vi "禹山浊度校准.vi"() -> ()   [LabVIEW 2016, in "斯坦道多参数.lvlib"]
uses:
  <vilib>/Utility/miscctls.llb/LVPointTypeDef.ctl
  <vilib>/Analysis/NI_AALBase.lvlib
  <vilib>/Analysis/NI_AALPro.lvlib
  <vilib>/Utility/config.llb/NI_LVConfig.lvlib
panel:
  out "第二点校准值":dbl
  out "第一点校准值":dbl
  out "最小值":sgl format="%.2g"
  out "最大值":sgl format="%.2g"
  in  "校准停止":bool
  in  "校准模式":enum16{"两点校准", "单点校准"}(ring)
  in  "标液2":dbl
  in  "标液1":dbl
  out "波形图表":sgl(graph) caption="历史曲线"
  out "温度测量值":dbl caption="温度"
  out "变异系数":dbl format="%.6g"
  out "standard deviation":dbl caption="标准差" format="%0.2f"
  out "mean":dbl caption="均值" format="%0.2f"
  out "提示":string
  in  "校准启动":bool
  out "测试值":dbl
  out "电极斜率":dbl
  out "电极零点":dbl
  # "浊度电极设定"
  # "℃"
  # "NTU"
  # "请选择校准模式:"
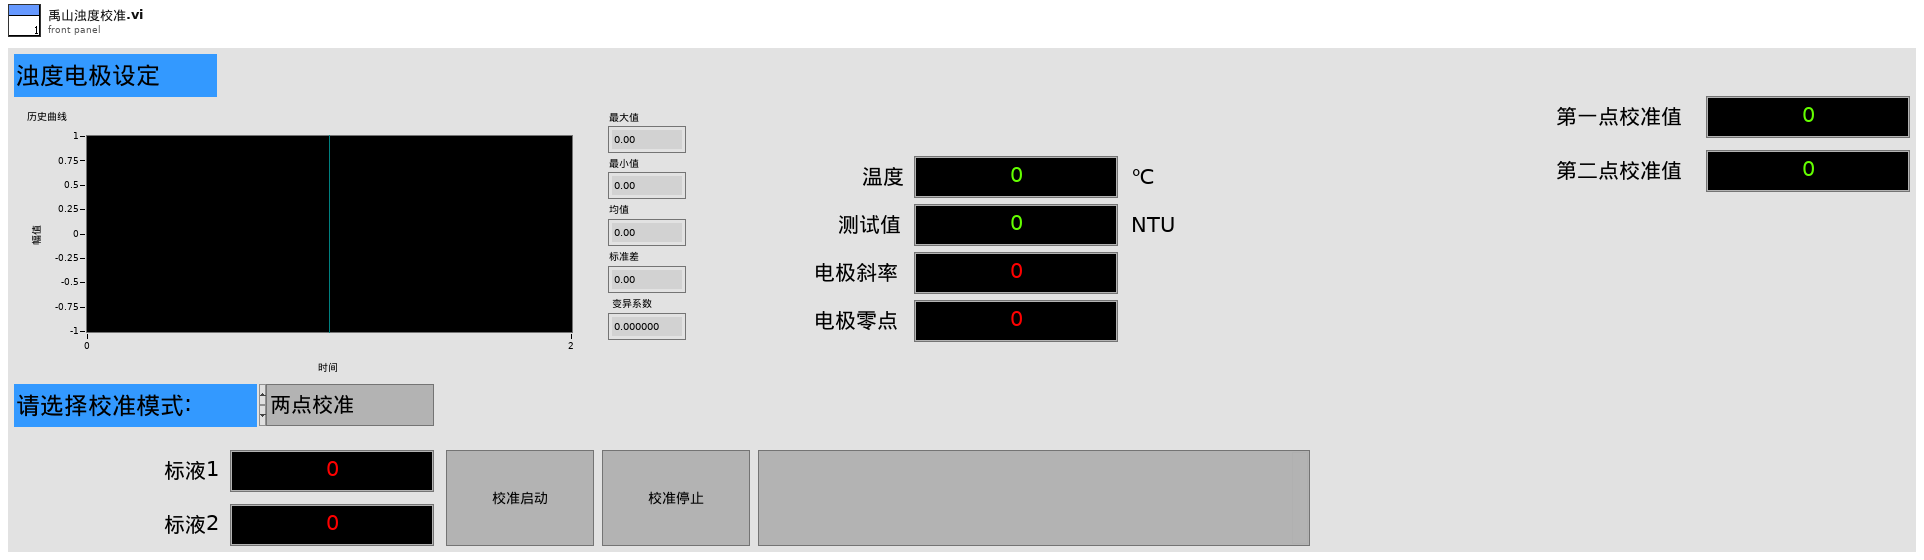
[diagram p1: front panel]
types:
  T1 = typedef "斯坦道多参数.lvlib/校准步骤.ctl" = enum16{"待机", "放置第一点标液", "第一点校准启动", "第一点校准写入", "第一点校准失败", "放置第二点标液", "第二点校准启动", "第二点校准写入", "第二点校准失败", "校准结果写入", "校准结束"}
  T2 = typedef "LVPointTypeDef.ctl" = cluster{"Horizontal":i16, "Vertical":i16}
  T3 = typedef "NI_LVConfig.lvlib/Config Data RefNum.ctl" = refnum<k1>
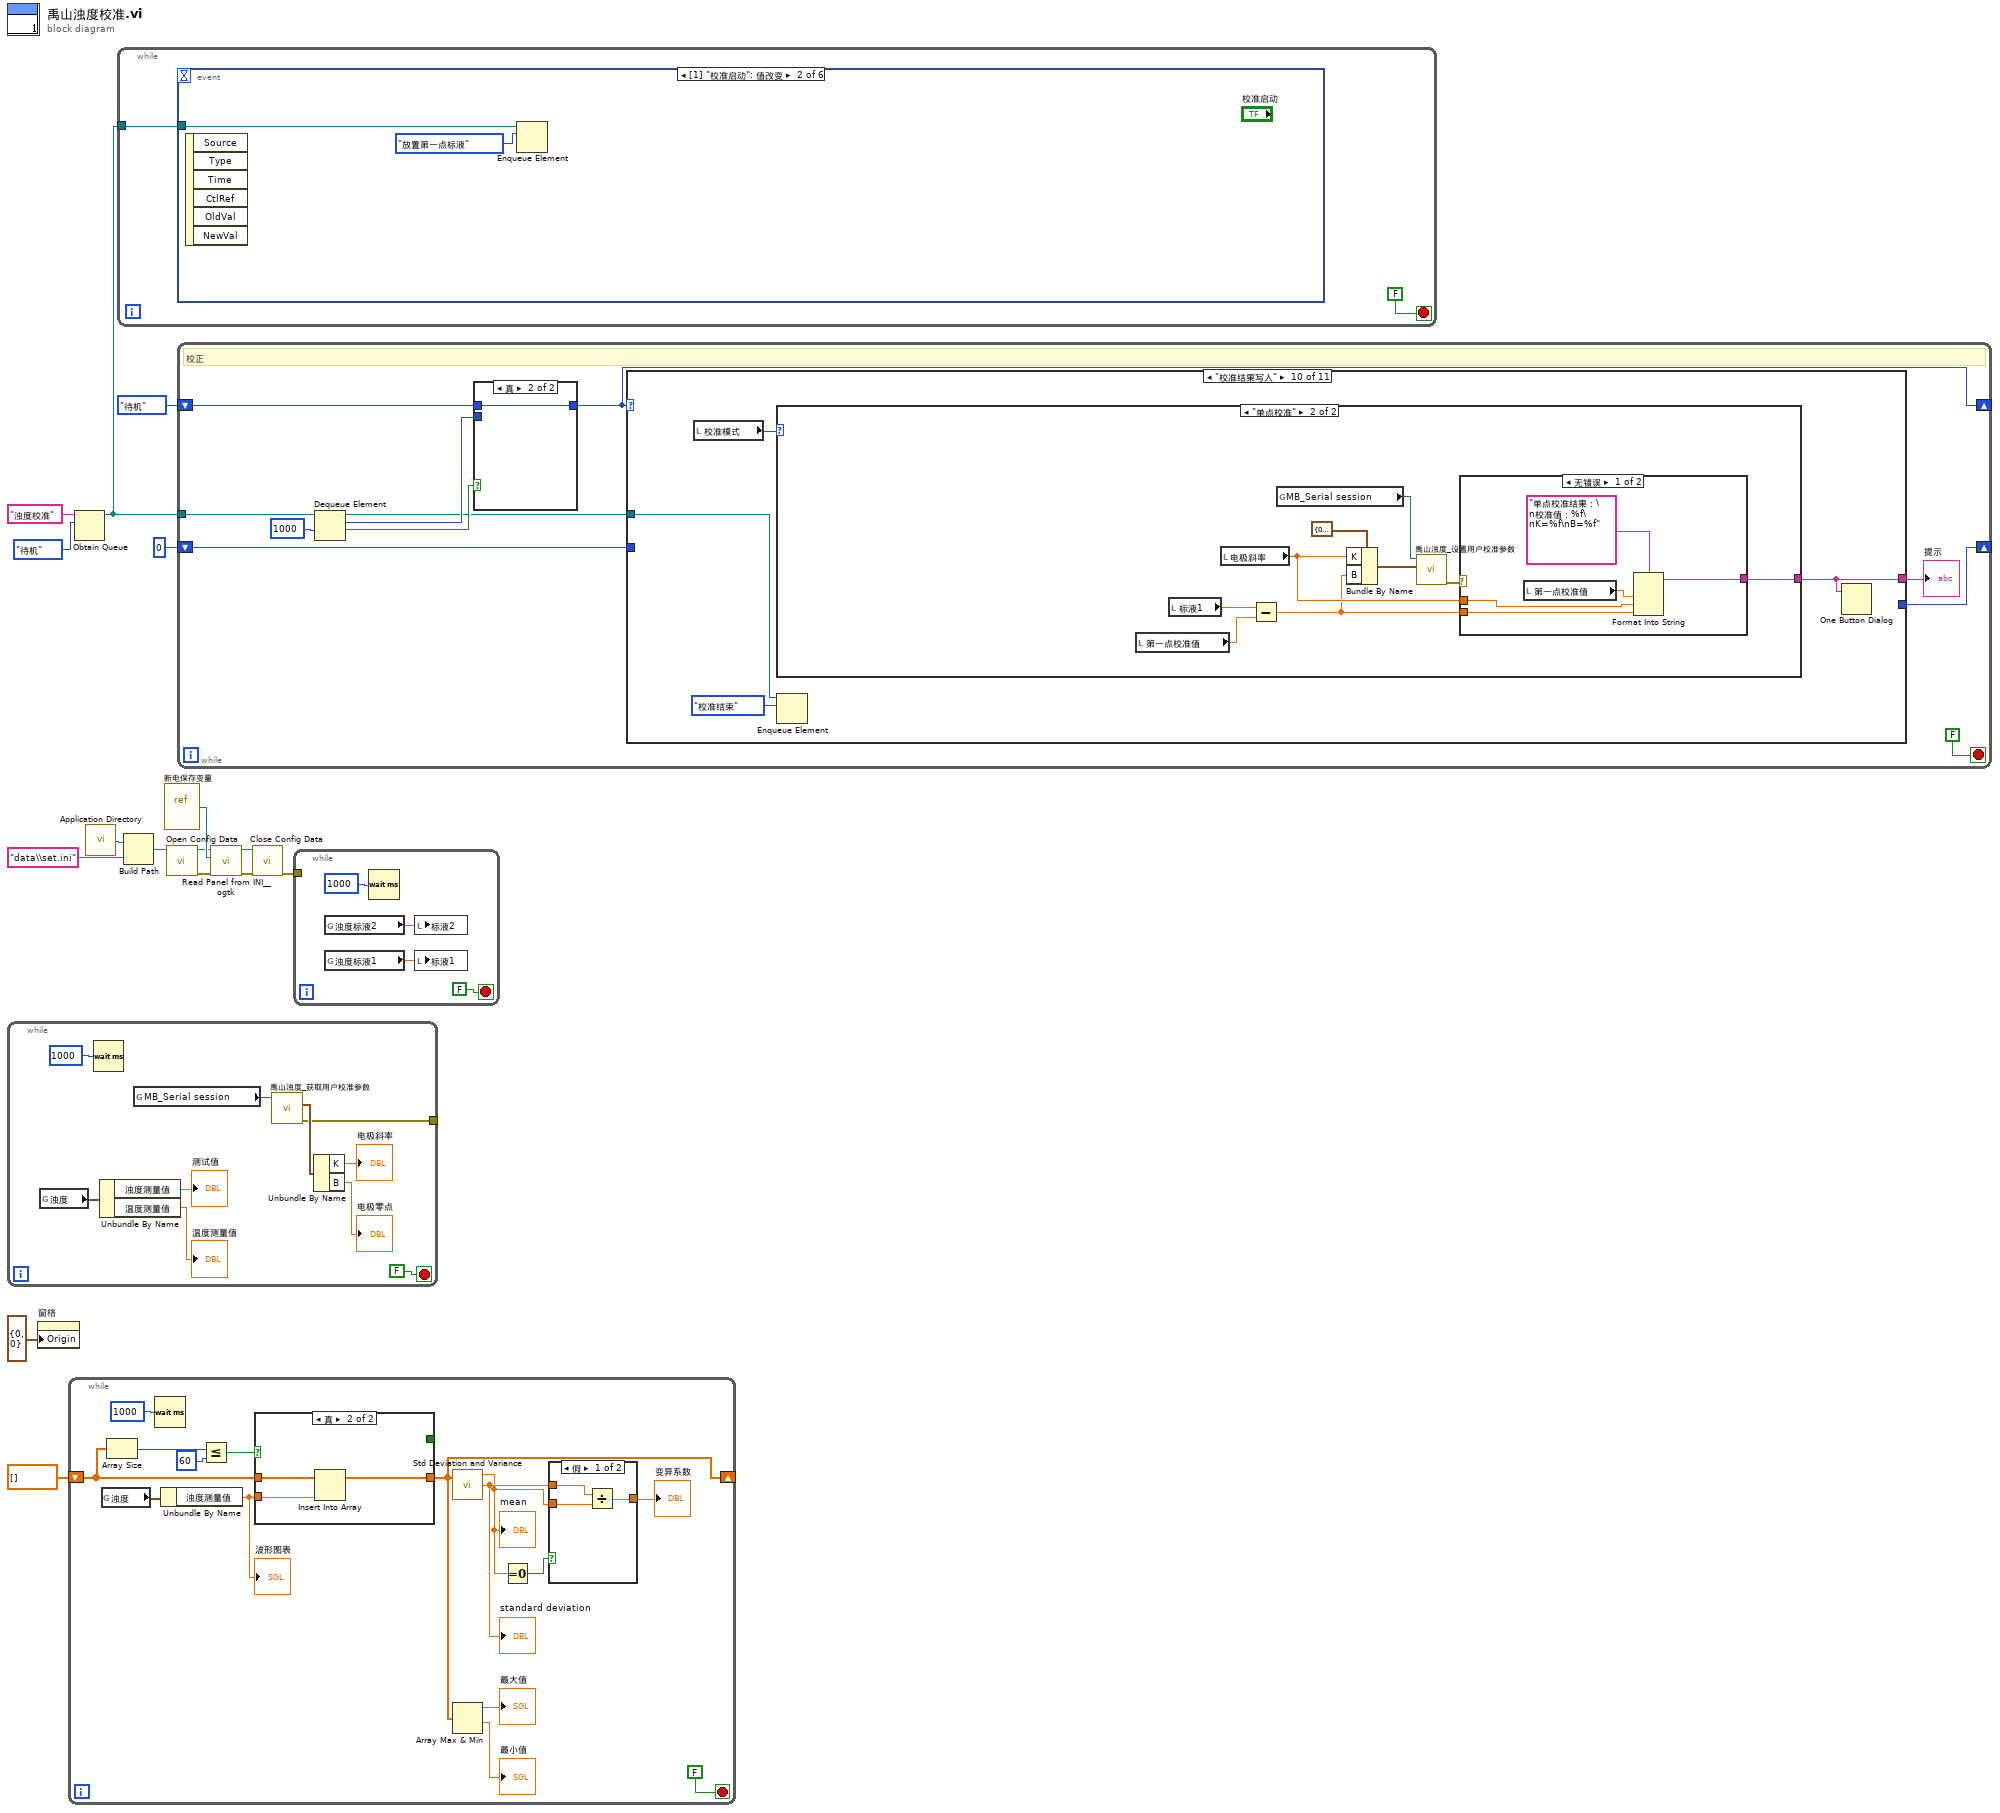
[diagram p0: block diagram]
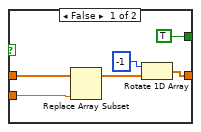
[diagram p3: hidden frame]
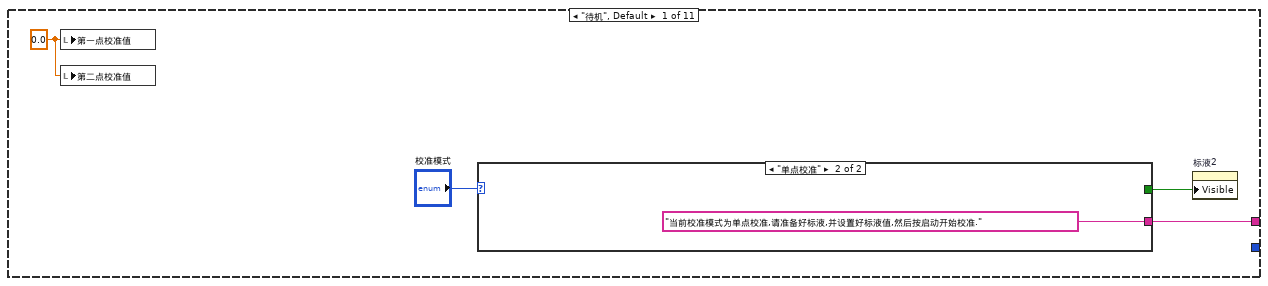
[diagram p5: hidden frame]
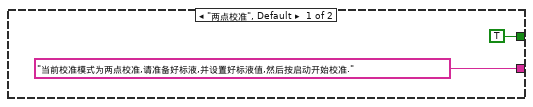
[diagram p6: hidden frame]
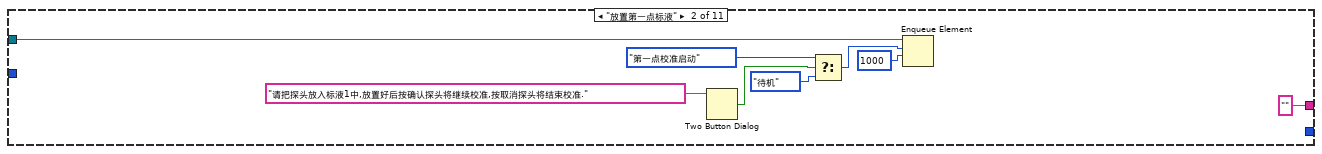
[diagram p7: hidden frame]
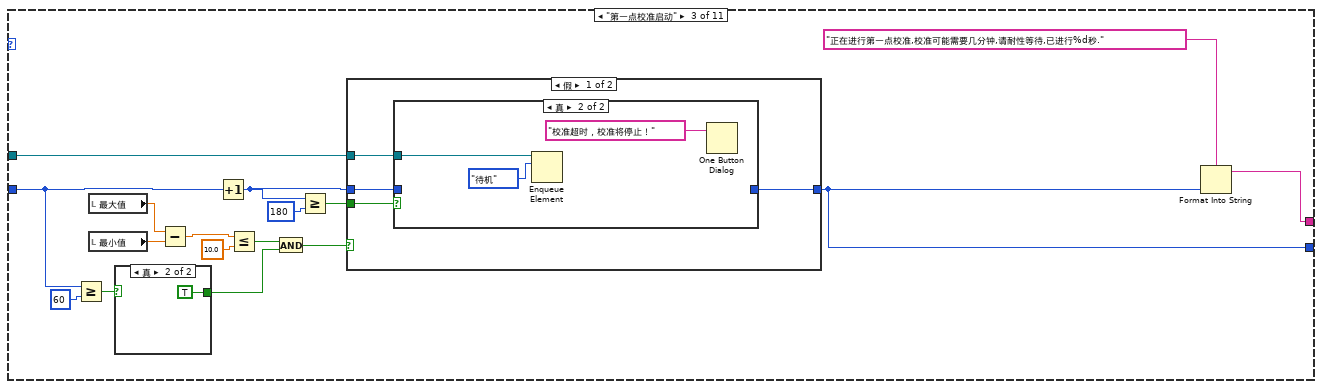
[diagram p8: hidden frame]
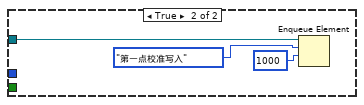
[diagram p10: hidden frame]
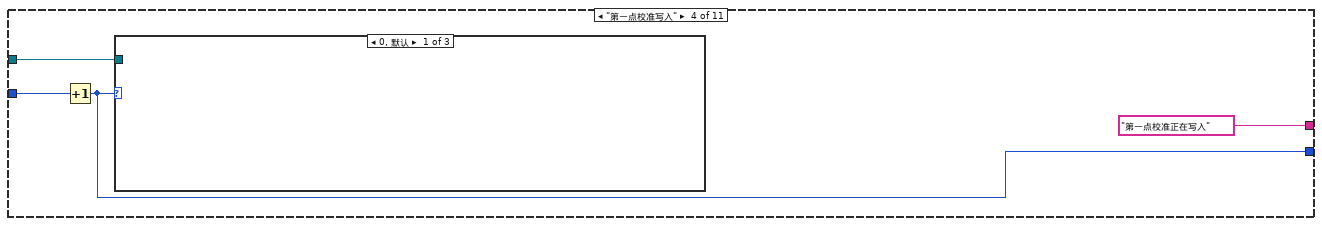
[diagram p12: hidden frame]
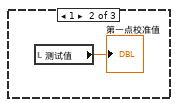
[diagram p13: hidden frame]
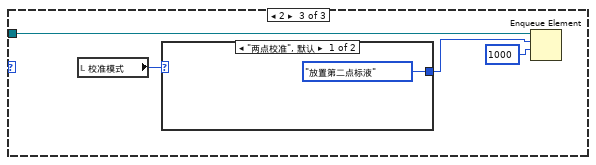
[diagram p14: hidden frame]
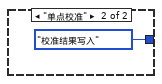
[diagram p15: hidden frame]
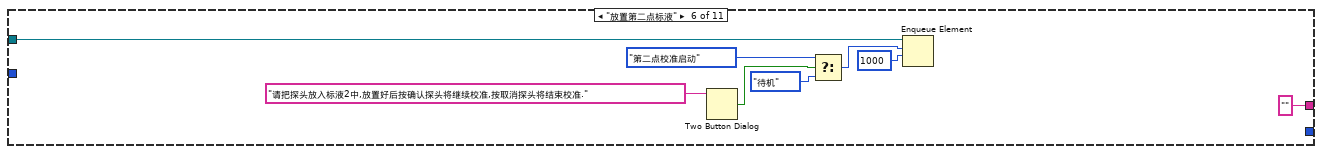
[diagram p17: hidden frame]
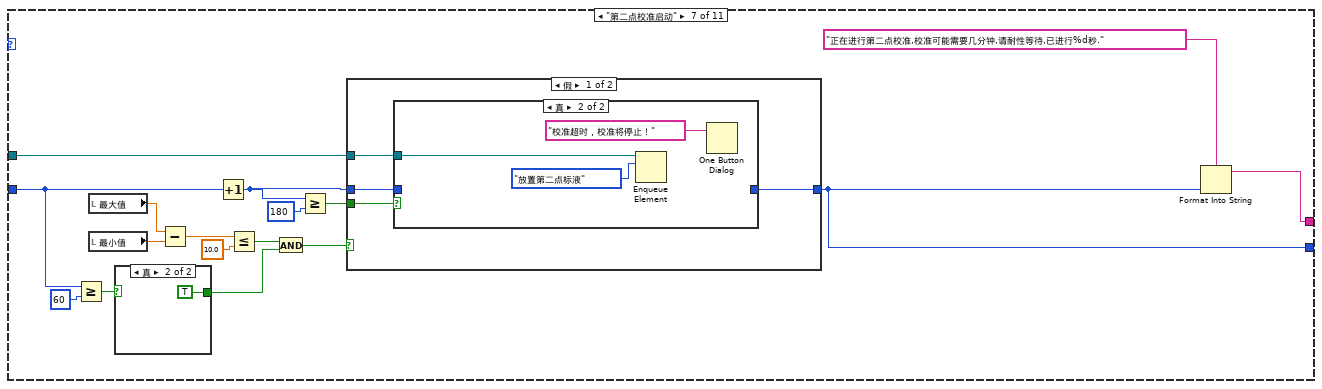
[diagram p18: hidden frame]
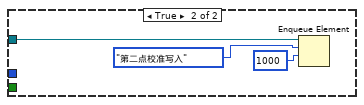
[diagram p20: hidden frame]
diagram:
  n1 = while {
    tunnel: [w21] -> _
    stop <- FALSE stop-if-true
    n2 = global read "禹山过程全局变量.vi" "浊度"() -> (w18:cluster{"温度测量值":sgl, "浊度测量值":sgl})
    n3 = Wait (ms)(milliseconds to wait=u32 1000 ("等待时间（毫秒）")) -> ()  [unwired: 1 out]
    n4 = Unbundle By Name(w18) -> ("浊度测量值"=→"测试值":sgl, "温度测量值"=→"温度测量值":sgl)
    n5 = global read "多参数全局变量.vi" "MB_Serial session"() -> (w17:refnum<class "MB_Master_Serial.lvclass">)
    n6 = call "禹山浊度_获取用户校准参数.vi"("MB_Serial session in"=w17) -> ("error out"=w21:errorcluster, "输出值"=w24:cluster{"K":sgl, "B":sgl})  [unwired: 8 in, 1 out]
    n7 = Unbundle By Name(w24) -> ("K"=→"电极斜率":sgl, "B"=→"电极零点":sgl)
  }
  n8 = property on="窗格" class="Pane"("Origin"=T2 {"Horizontal"=0, "Vertical"=0} ("原点")) -> ()  [unwired: 2 in, 2 out]
  n9 = while {
    shift-right: [w29] -> _
    shift-left: sgl[] [] -> [w37]
    stop <- FALSE stop-if-true
    n10 = global read "禹山过程全局变量.vi" "浊度"() -> (w31:cluster{"温度测量值":sgl, "浊度测量值":sgl})
    n11 = Array Size(array=w37) -> (size(s)=w39:i32)
    n12 = Wait (ms)(milliseconds to wait=u32 1000 ("等待时间（毫秒）")) -> ()  [unwired: 1 out]
    n13 = Unbundle By Name(w31) -> ("浊度测量值"=w30:sgl)
    "波形图表" <- w30
    n14 = Less Or Equal?(x=w39, y=60) -> (x <= y?=w38:bool)
    n15 = case shown="真" w38 {
      tunnel: w37 -> [w50 w53]
      tunnel: w30 -> [w48 w52]
      tunnel: [w46 w51] -> w29
      tunnel: [TRUE _] -> _
      frame False {
        n16 = Replace Array Subset(array=w50, new element=w48) -> (w49:sgl[])  [unwired: 1 in]
        n17 = Rotate 1D Array(1:w49, 2:-1 ("n")) -> (0:w46:sgl[])
      }
      frame True {
        n18 = Insert Into Array(array=w53, new element=w52) -> (w51:sgl[])  [unwired: 1 in]
      }
    }
    n19 = call <vilib>:"Std Deviation and Variance.vi"("X"=w29) -> ("mean"=w32:dbl, "standard deviation"=w33:dbl)  [unwired: 1 in, 1 out]
    "standard deviation" <- w33
    "mean" <- w32
    n20 = Array Max & Min(array=w29) -> (max value=→"最大值":sgl, min value=→"最小值":sgl)  [unwired: 2 out]
    n21 = Equal To 0?(x=w32) -> (x = 0?=w36:bool)
    n22 = case shown="假" w36 {
      tunnel: w33 -> [w44 _]
      tunnel: [w43 _] -> w35
      tunnel: w32 -> [w42 _]
      frame False {
        n23 = Divide(x=w44, y=w42) -> (x/y=w43:dbl)
      }
      frame True {
      }
    }
    "变异系数" <- w35
  }
  n24 = Obtain Queue(name (unnamed)="浊度校准" ("名称（未命名）"), element data type=校准步骤."待机" ("枚举")) -> (queue out=w10:refnum<queue>)  [unwired: 3 in, 2 out]
  n25 = call <vilib>:"Application Directory.vi"() -> ("Application Directory"=w6:path)
  n26 = while {
    tunnel: w10 -> [w54]
    stop <- FALSE stop-if-true
    n27 = event shown="[1] \"校准启动\": 值改变" {
      selector: _ -> [_ _ _ _ _ _]
      dyn-events: _ -> [_ _ _ _ _ _]
      timeout: _ -> [_ _ _ _ _ _]
      tunnel: w54 -> [_ w57 w61 _ _ _]
      event Timeout {
        n28 = event-data() -> ()  [unwired: 1 in, 3 out]
      }
      event "校准启动": Value Change {
        n29 = event-data() -> ()  [unwired: 1 in, 6 out]
        n30 = Enqueue Element(queue=w57, element=校准步骤."放置第一点标液" ("元素")) -> ()  [unwired: 2 in, 3 out]
      }
      event "校准停止": Value Change {
        n31 = event-data() -> ()  [unwired: 1 in, 6 out]
        n32 = Flush Queue(queue=w61) -> (queue out=w58:refnum<queue>)  [unwired: 1 in, 2 out]
        n33 = Enqueue Element(queue=w58, element=校准步骤."待机" ("元素"), timeout in ms (-1)=1000 ("超时毫秒(-1)")) -> ()  [unwired: 1 in, 3 out]
      }
      event "电极零点", "电极斜率", "标液1", "标液2": Mouse Down {
        n34 = event-data() -> ("CtlRef"=w62:refnum<vi>)  [unwired: 1 in, 7 out]
        n35 = property class="DigNum (严格)"(reference=w62) -> (reference out=w63:refnum<vi>, "Value"=w64:dbl)  [unwired: 1 in, 1 out]
        n36 = call "数字键盘.vi"("OldNumber"=w64) -> ("NewNumber"=w65:sgl)
        n37 = property class="DigNum (严格)"(reference=w63, "Val(Sgnl)"=w65) -> ()  [unwired: 1 in, 2 out]
      }
      event "电极零点", "电极斜率": Value Change {
        n38 = event-data() -> ()  [unwired: 1 in, 6 out]
        n39 = local read "电极斜率"() -> (w68:dbl)
        n40 = local read "电极零点"() -> (w67:dbl)
        n41 = global read "多参数全局变量.vi" "MB_Serial session"() -> (w66:refnum<class "MB_Master_Serial.lvclass">)
        n42 = Bundle By Name(cluster=cluster{"K":sgl, "B":sgl} {"K"=0.0, "B"=0.0} ("用户校准参数"), "K"=w68, "B"=w67) -> (w69:cluster{"K":sgl, "B":sgl})
        n43 = call "禹山浊度_设置用户校准参数.vi"("用户校准参数"=w69, "MB_Serial session in"=w66) -> ()  [unwired: 8 in, 2 out]
      }
      event "标液1", "标液2": Value Change {
        n44 = event-data() -> ()  [unwired: 1 in, 6 out]
        n45 = flat-sequence {
          frame #0 {
            n46 = global write "断电保存变量.vi" "浊度标液2"("标液2") -> ()
            n47 = global write "断电保存变量.vi" "浊度标液1"("标液1") -> ()
          }
          frame #1 {
            n48 = call <vilib>:"Application Directory.vi"() -> ("Application Directory"=w82:path)
            n49 = Build Path(base path=w82, name or relative path="data\\set.ini" ("名称或相对路径")) -> (appended path=w81:path)
            n50 = call <vilib>:"Open Config Data.vi"("configuration file path"=w81) -> ("error out"=w85:errorcluster, "refnum"=w86:T3)  [unwired: 8 in, 1 out]
            n51 = vi-ref "断电保存变量.vi"() -> (w79:refnum<vi>)
            n52 = call <userlib>:"Write Panel to INI__ogtk.vi"("error in (no error)"=w85, "VI ref"=w79, "refnum"=w86) -> ("error out"=w83:errorcluster, "refnum out"=w84:T3)  [unwired: 7 in]
            n53 = call <vilib>:"Close Config Data.vi"("error in (no error)"=w83, "refnum"=w84) -> ("error out"=w75:errorcluster, "file path"=w76:path)  [unwired: 8 in]
            n54 = Open/Create/Replace File(file path (use dialog)=w76, error in=w75) -> (refnum out=w77:refnum<file>, error out=w78:errorcluster)  [unwired: 4 in, 1 out]
            n55 = Flush File(refnum=w77, error in=w78) -> (refnum out=w73:refnum<file>, error out=w74:errorcluster)
            n56 = Close File(refnum=w73, error in=w74) -> ()  [unwired: 2 out]
          }
        }
      }
    }
  }
  n57 = Build Path(base path=w6, name or relative path="data\\set.ini" ("名称或相对路径")) -> (appended path=w7:path)
  n58 = vi-ref "断电保存变量.vi"() -> (w9:refnum<vi>)
  n59 = call <vilib>:"Open Config Data.vi"("configuration file path"=w7) -> ("error out"=w3:errorcluster, "refnum"=w2:T3)  [unwired: 8 in, 1 out]
  n60 = while "While循环" {
    shift-right: [w88] -> _
    shift-left: 校准步骤."待机" ("枚举") -> [w89]
    shift-right: [w95] -> _
    shift-left: 0 -> [w96]
    tunnel: w10 -> [w93]
    stop <- FALSE stop-if-true
    # "校正"
    n61 = Dequeue Element(queue=w93, timeout in ms (-1)=1000 ("超时毫秒(-1)")) -> (queue out=w87:refnum<queue>, element=w90:T1, timed out?=w91:bool)  [unwired: 1 in, 1 out]
    n62 = case shown="真" w91 {
      tunnel: w90 -> [w98 _]
      tunnel: [w98 w99] -> w88
      tunnel: w89 -> [_ w99]
      frame False {
      }
      frame True {
      }
    }
    n63 = case shown="\"校准结果写入\"" w88 {
      tunnel: [w103 "" ("提示") w130 "第一点校准正在写入" ("提示") _ "" ("提示") w178 "第二点校准正在写入" ("提示") _ w203 w246] -> w94
      tunnel: w96 -> [_ _ w124 w146 _ _ w172 w194 _ _ _]
      tunnel: [_ _ w115 w145 _ _ w163 w193 _ _ _] -> w95
      tunnel: w87 -> [_ w113 w118 w144 _ w161 w166 w192 _ w202 _]
      frame "待机", Default {
        w100 = 0.0 ("第一点校准值")
        n64 = local write "第一点校准值"(w100) -> ()
        n65 = local write "第二点校准值"(w100) -> ()
        n66 = case shown="\"单点校准\"" "校准模式" {
          tunnel: ["当前校准模式为两点校准,请准备好标液,并设置好标液值,然后按启动开始校准." ("提示") "当前校准模式为单点校准,请准备好标液,并设置好标液值,然后按启动开始校准." ("提示")] -> w103
          tunnel: [TRUE ("可见") _] -> w101
          frame "两点校准", Default {
          }
          frame "单点校准" {
          }
        }
        n67 = property on="标液2" class="DigNum (严格)"("Visible"=w101) -> ()  [unwired: 2 in, 2 out]
      }
      frame "放置第一点标液" {
        n68 = Two Button Dialog(message="请把探头放入标液1中,放置好后按确认探头将继续校准,按取消探头将结束校准." ("消息")) -> (T button?=w111:bool)  [unwired: 2 in]
        n69 = Select(t=校准步骤."第一点校准启动" ("元素"), s=w111, f=校准步骤."待机" ("元素")) -> (s? t:f=w108:T1)
        n70 = Enqueue Element(queue=w113, element=w108, timeout in ms (-1)=1000 ("超时毫秒(-1)")) -> ()  [unwired: 1 in, 3 out]
      }
      frame "第一点校准启动" {
        n71 = Greater Or Equal?(x=w124, y=60) -> (x >= y?=w125:bool)
        n72 = local read "最大值"() -> (w121:sgl)
        n73 = local read "最小值"() -> (w122:sgl)
        n74 = case shown="真" w125 {
          tunnel: [_ TRUE] -> w123
          frame False {
          }
          frame True {
          }
        }
        n75 = Subtract(x=w121, y=w122) -> (x-y=w120:sgl)
        n76 = Increment(x=w124) -> (x+1=w116:i32)
        n77 = Less Or Equal?(x=w120, y=10.0) -> (x <= y?=w128:bool)
        n78 = And(x=w128, y=w123) -> (x .and. y?=w119:bool)
        n79 = Greater Or Equal?(x=w116, y=180) -> (x >= y?=w117:bool)
        n80 = case shown="假" w119 {
          tunnel: w118 -> [w134 w142]
          tunnel: w117 -> [w135 _]
          tunnel: w116 -> [w133 _]
          tunnel: [w132 _] -> w115
          frame False {
            n81 = case shown="真" w135 {
              tunnel: w134 -> [_ w139]
              tunnel: w133 -> [w136 _]
              tunnel: [w136 _] -> w132
              frame False {
              }
              frame True {
                n82 = Enqueue Element(queue=w139, element=校准步骤."待机" ("元素")) -> ()  [unwired: 2 in, 3 out]
                n83 = One Button Dialog(message="校准超时，校准将停止！" ("消息")) -> ()  [unwired: 1 in, 1 out]
              }
            }
          }
          frame True {
            n84 = Enqueue Element(queue=w142, element=校准步骤."第一点校准写入" ("元素"), timeout in ms (-1)=1000 ("超时毫秒(-1)")) -> ()  [unwired: 1 in, 3 out]
          }
        }
        n85 = Format Into String(format string="正在进行第一点校准,校准可能需要几分钟,请耐性等待,已进行%d秒." ("格式字符串"), w115) -> (resulting string=w130:string)  [unwired: 2 in, 1 out]
      }
      frame "第一点校准写入" {
        n86 = Increment(x=w146) -> (x+1=w145:i32)
        n87 = case shown="0, 默认" w145 {
          tunnel: w144 -> [_ _ w152]
          frame 0, Default {
          }
          frame 1 {
            n88 = local read "测试值"() -> (→"第一点校准值":dbl)
          }
          frame 2 {
            n89 = local read "校准模式"() -> (w151:enum16{"两点校准", "单点校准"})
            n90 = case shown="\"两点校准\", 默认" w151 {
              tunnel: [校准步骤."放置第二点标液" ("元素") 校准步骤."校准结果写入" ("元素")] -> w150
              frame "两点校准", Default {
              }
              frame "单点校准" {
              }
            }
            n91 = Enqueue Element(queue=w152, element=w150, timeout in ms (-1)=1000 ("超时毫秒(-1)")) -> ()  [unwired: 1 in, 3 out]
          }
        }
      }
      frame "第一点校准失败" {
      }
      frame "放置第二点标液" {
        n92 = Two Button Dialog(message="请把探头放入标液2中,放置好后按确认探头将继续校准,按取消探头将结束校准." ("消息")) -> (T button?=w159:bool)  [unwired: 2 in]
        n93 = Select(t=校准步骤."第二点校准启动" ("元素"), s=w159, f=校准步骤."待机" ("元素")) -> (s? t:f=w156:T1)
        n94 = Enqueue Element(queue=w161, element=w156, timeout in ms (-1)=1000 ("超时毫秒(-1)")) -> ()  [unwired: 1 in, 3 out]
      }
      frame "第二点校准启动" {
        n95 = Greater Or Equal?(x=w172, y=60) -> (x >= y?=w173:bool)
        n96 = local read "最大值"() -> (w169:sgl)
        n97 = local read "最小值"() -> (w170:sgl)
        n98 = case shown="真" w173 {
          tunnel: [_ TRUE] -> w171
          frame False {
          }
          frame True {
          }
        }
        n99 = Subtract(x=w169, y=w170) -> (x-y=w168:sgl)
        n100 = Increment(x=w172) -> (x+1=w164:i32)
        n101 = Less Or Equal?(x=w168, y=10.0) -> (x <= y?=w176:bool)
        n102 = And(x=w176, y=w171) -> (x .and. y?=w167:bool)
        n103 = Greater Or Equal?(x=w164, y=180) -> (x >= y?=w165:bool)
        n104 = case shown="假" w167 {
          tunnel: w166 -> [w182 w190]
          tunnel: w165 -> [w183 _]
          tunnel: w164 -> [w181 _]
          tunnel: [w180 _] -> w163
          frame False {
            n105 = case shown="真" w183 {
              tunnel: w182 -> [_ w187]
              tunnel: w181 -> [w184 _]
              tunnel: [w184 _] -> w180
              frame False {
              }
              frame True {
                n106 = Enqueue Element(queue=w187, element=校准步骤."放置第二点标液" ("元素")) -> ()  [unwired: 2 in, 3 out]
                n107 = One Button Dialog(message="校准超时，校准将停止！" ("消息")) -> ()  [unwired: 1 in, 1 out]
              }
            }
          }
          frame True {
            n108 = Enqueue Element(queue=w190, element=校准步骤."第二点校准写入" ("元素"), timeout in ms (-1)=1000 ("超时毫秒(-1)")) -> ()  [unwired: 1 in, 3 out]
          }
        }
        n109 = Format Into String(format string="正在进行第二点校准,校准可能需要几分钟,请耐性等待,已进行%d秒." ("格式字符串"), w163) -> (resulting string=w178:string)  [unwired: 2 in, 1 out]
      }
      frame "第二点校准写入" {
        n110 = Increment(x=w194) -> (x+1=w193:i32)
        n111 = case shown="2" w193 {
          tunnel: w192 -> [_ _ w199]
          frame 0, Default {
          }
          frame 1 {
            n112 = local read "测试值"() -> (→"第二点校准值":dbl)
          }
          frame 2 {
            n113 = Enqueue Element(queue=w199, element=校准步骤."校准结果写入" ("元素"), timeout in ms (-1)=1000 ("超时毫秒(-1)")) -> ()  [unwired: 1 in, 3 out]
          }
        }
      }
      frame "第二点校准失败" {
      }
      frame "校准结果写入" {
        n114 = local read "校准模式"() -> (w200:enum16{"两点校准", "单点校准"})
        n115 = case shown="\"单点校准\"" w200 {
          tunnel: [w211 w235] -> w203
          frame "两点校准", Default {
            n116 = local read "第一点校准值"() -> (w222:dbl)
            n117 = local read "第二点校准值"() -> (w221:dbl)
            n118 = local read "标液1"() -> (w219:dbl)
            n119 = local read "标液2"() -> (w218:dbl)
            n120 = Insert Into Array(array=dbl[] [] ("Weight"), new element #1=w219, new element #2=w218) -> (w217:dbl[])  [unwired: 1 in]
            n121 = Insert Into Array(array=dbl[] [] ("Weight"), new element #1=w222, new element #2=w221) -> (w216:dbl[])  [unwired: 1 in]
            n122 = local read "电极零点"() -> (w207:dbl)
            n123 = call <vilib>:"Linear Fit.vi"("Y"=w217, "X"=w216) -> ("slope"=w208:dbl, "intercept"=w205:dbl)  [unwired: 9 in, 3 out]
            n124 = local read "电极斜率"() -> (w210:dbl)
            n125 = Multiply(x=w208, y=w207) -> (x*y=w206:dbl)
            n126 = Multiply(x=w210, y=w208) -> (x*y=w209:dbl)
            n127 = Add(x=w206, y=w205) -> (x+y=w204:dbl)
            n128 = global read "多参数全局变量.vi" "MB_Serial session"() -> (w215:refnum<class "MB_Master_Serial.lvclass">)
            n129 = Bundle By Name(cluster=cluster{"K":sgl, "B":sgl} {"K"=0.0, "B"=0.0} ("用户校准参数"), "K"=w209, "B"=w204) -> (w214:cluster{"K":sgl, "B":sgl})
            n130 = call "禹山浊度_设置用户校准参数.vi"("用户校准参数"=w214, "MB_Serial session in"=w215) -> ("error out"=w212:errorcluster)  [unwired: 8 in, 1 out]
            n131 = case shown="无错误" w212 {
              tunnel: w209 -> [w226 _]
              tunnel: w204 -> [w225 _]
              tunnel: [w224 "校准失败"] -> w211
              frame No Error {
                n132 = local read "第一点校准值"() -> (w228:dbl)
                n133 = local read "第二点校准值"() -> (w229:dbl)
                n134 = Format Into String(format string="两点校准结果：\n第一点校准值：%f\n第二点校准值：%f\nK=%f\nB=%f" ("提示"), w228, w229, w226, w225) -> (resulting string=w224:string)  [unwired: 2 in, 1 out]
              }
              frame Error {
              }
            }
          }
          frame "单点校准" {
            n135 = local read "第一点校准值"() -> (w233:dbl)
            n136 = local read "标液1"() -> (w232:dbl)
            n137 = local read "电极斜率"() -> (w234:dbl)
            n138 = Subtract(x=w232, y=w233) -> (x-y=w231:dbl)
            n139 = global read "多参数全局变量.vi" "MB_Serial session"() -> (w239:refnum<class "MB_Master_Serial.lvclass">)
            n140 = Bundle By Name(cluster=cluster{"K":sgl, "B":sgl} {"K"=0.0, "B"=0.0} ("用户校准参数"), "K"=w234, "B"=w231) -> (w238:cluster{"K":sgl, "B":sgl})
            n141 = call "禹山浊度_设置用户校准参数.vi"("用户校准参数"=w238, "MB_Serial session in"=w239) -> ("error out"=w236:errorcluster)  [unwired: 8 in, 1 out]
            n142 = case shown="无错误" w236 {
              tunnel: w234 -> [w242 _]
              tunnel: w231 -> [w241 _]
              tunnel: [w240 "校准失败"] -> w235
              frame No Error {
                n143 = local read "第一点校准值"() -> (w244:dbl)
                n144 = Format Into String(format string="单点校准结果：\n校准值：%f\nK=%f\nB=%f" ("提示"), w244, w242, w241) -> (resulting string=w240:string)  [unwired: 2 in, 1 out]
              }
              frame Error {
              }
            }
          }
        }
        n145 = Enqueue Element(queue=w202, element=校准步骤."校准结束" ("元素")) -> ()  [unwired: 2 in, 3 out]
        n146 = One Button Dialog(message=w203) -> ()  [unwired: 1 in, 1 out]
      }
      frame "校准结束" {
        n147 = local read "提示"() -> (w246:string)
      }
    }
    "提示" <- w94
  }
  n148 = call <userlib>:"Read Panel from INI__ogtk.vi"("error in (no error)"=w3, "VI ref"=w9, "refnum"=w2) -> ("error out"=w5:errorcluster, "refnum out"=w4:T3)  [unwired: 7 in]
  n149 = call <vilib>:"Close Config Data.vi"("error in (no error)"=w5, "refnum"=w4) -> ("error out"=w1:errorcluster)  [unwired: 8 in, 1 out]
  n150 = while {
    tunnel: w1 -> [_]
    stop <- FALSE stop-if-true
    n151 = global read "断电保存变量.vi" "浊度标液2"() -> (w247:dbl)
    n152 = global read "断电保存变量.vi" "浊度标液1"() -> (w248:dbl)
    n153 = Wait (ms)(milliseconds to wait=u32 1000 ("等待时间（毫秒）")) -> ()  [unwired: 1 out]
    n154 = local write "标液2"(w247) -> ()
    n155 = local write "标液1"(w248) -> ()
  }
